vi "WritePort.vi"(0 "NXP in":refnum<class "NXP.lvclass">, 5 "VISA resource name":refnum<visa-resource-name>, 7 "Puerto":u8, 9 "Array":bool[](array[boolean]), 11 "error in (no error)":errorcluster) -> (4 "NXP out":refnum<class "NXP.lvclass">, 6 "VISA resource name 2":refnum<visa-resource-name>, 8 "Expected command":string, 15 "error out":errorcluster)   [LabVIEW 2020, in "NXP.lvclass"]
doc: "Write Port NXP. \nSe encarga de escribir un puerto completo por VISA, mandando un arreglo de boleanos de modo serial y obteniendo el mismo arreglo en los leds de su NXP"
uses:
  NXP.lvclass
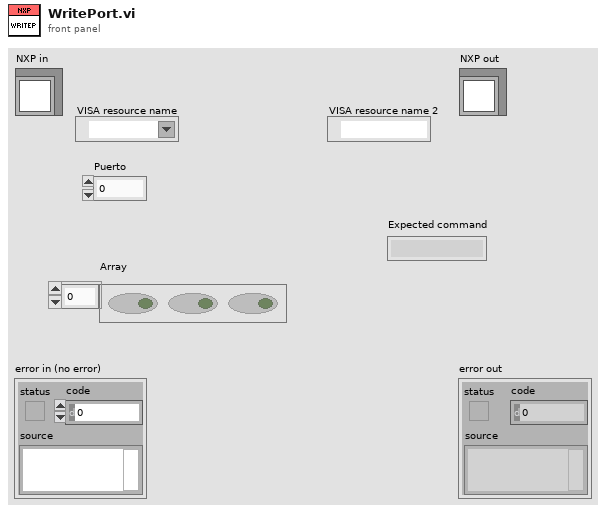
[diagram p1: front panel]
types:
  T1 = enum16{"Write", "Read", "Config", "Reset", "Close"}
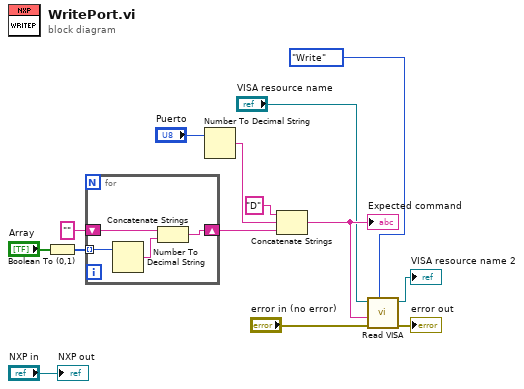
[diagram p0: block diagram]
diagram:
  n1 = Boolean To (0,1)(Boolean="Array") -> (0, 1=w12:i16[])
  n2 = for {
    tunnel: w12 -> [w18] mode=indexing
    shift-right: [w16] -> w7
    shift-left: "" -> [w15]
    n3 = Number To Decimal String(number=w18) -> (decimal integer string=w17:string)  [unwired: 1 in]
    n4 = Concatenate Strings(w15, w17) -> (w16:string)
  }
  n5 = Number To Decimal String(number="Puerto") -> (decimal integer string=w8:string)  [unwired: 1 in]
  n6 = Concatenate Strings("D" ("string"), w8, w7) -> (w5:string)
  "Expected command" <- w5
  n7 = call "Read VISA.vi"("Opciones"=T1."Write", "error in (no error)"="error in (no error)", "Write"=w5, "VISA com port"="VISA resource name") -> ("error out"=→"error out":errorcluster, "VISA com port 2"=→"VISA resource name 2":refnum<visa-resource-name>)  [unwired: 5 in, 1 out]
  "NXP out" <- "NXP in"
